vi "Scan Calculations.vi"(0 "counter cluster in":T6, 1 "control flags in":T5, 2 "N spot tracker in":T2, 3 "scan specification in":T7={"z resolution (pixels)"=1000, "iterations per pixel"=28, "iterations per z-scan (=zres*iterperpixel)"=50, "x resolution (pixels)"=100, "y resolution (pixels)"=80, "number of z-lines per volume"=30, "number of repetitions (volumes)"=5, "Pockels cell voltage (bits)"=-1, "Vx center (bits)"=0, "Vy center (bits)"=0, "Vx amplitude (bits)"=40, "Vy amplitude (bits)"=0, "lines to delay between scan start and output"=1, "LSB has acquire control"=FALSE}, 4 "tracking settings":T9, 5 "3-axis PV tracking state in":T3, 6 "x-y phase shift (*2^16/2*pi)":u16=16384, 7 "min photons for update":u32=200, 8 "Tracking State Initializer":T1, 11 "stim buffer counts":u16=20) -> (10 "end scan":bool, 12 "trigger out":bool, 13 "kalman to host":cluster{"Kalman State":T4, "Kalman Update":bool}, 14 "counter cluster out":T6, 15 "control flags out":T5, 16 "N spot tracker out":T2, 17 "scan specification out":T7, 18 "DAC voltages":T8 {"pockels" max=4095 step=1; "y" max=4095 step=1; "x" max=4095 step=1}, 19 "3-axis PV tracking state out":T3={"x state"={"pos estimate"=0.0, "v estimate"=0.0, "weighted position error sum"=0.0, "photon count"=0, "transmit tick count"=0, "axis number"=0, "px (levels^2)"=0.0, "pxv (levels^2/ticks)"=0.0, "pv (levels^2/ticks^2)"=0.0, "vel diff (levels^2/ticks^3)"=0.0, "gx"=0.0, "rtwiddle"=0.0, "photon count ch0"=0, "photon count ch1"=0, "Dx - for pos only k-f"=0.0}, "y state"={"pos estimate"=0.0, "v estimate"=0.0, "weighted position error sum"=0.0, "photon count"=0, "transmit tick count"=0, "axis number"=1, "px (levels^2)"=0.0, "pxv (levels^2/ticks)"=0.0, "pv (levels^2/ticks^2)"=0.0, "vel diff (levels^2/ticks^3)"=0.0, "gx"=0.0, "rtwiddle"=0.0, "photon count ch0"=0, "photon count ch1"=0, "Dx - for pos only k-f"=0.0}, "z state"={"pos estimate"=0.0, "v estimate"=0.0, "weighted position error sum"=0.0, "photon count"=0, "transmit tick count"=0, "axis number"=2, "px (levels^2)"=0.0, "pxv (levels^2/ticks)"=0.0, "pv (levels^2/ticks^2)"=0.0, "vel diff (levels^2/ticks^3)"=0.0, "gx"=0.0, "rtwiddle"=0.0, "photon count ch0"=0, "photon count ch1"=0, "Dx - for pos only k-f"=0.0}})   [LabVIEW 2010]
uses:
  FPGA tracking/polar tracking settings.ctl
  common_typedefs/DAC_voltage_tagResonantr.ctl
  scan_specification_tagResonant.ctl
  counter_cluster_tagResonant.ctl
  FPGA tracking/kalman 3-axis state.ctl
  FPGA tracking/integrating single axis kalman state.ctl
  FPGA tracking/control flags.ctl
  FPGA tracking/kalman N spot state.ctl
  FPGA tracking/tracking state initializer.ctl
panel:
  out "checked out state number":u16
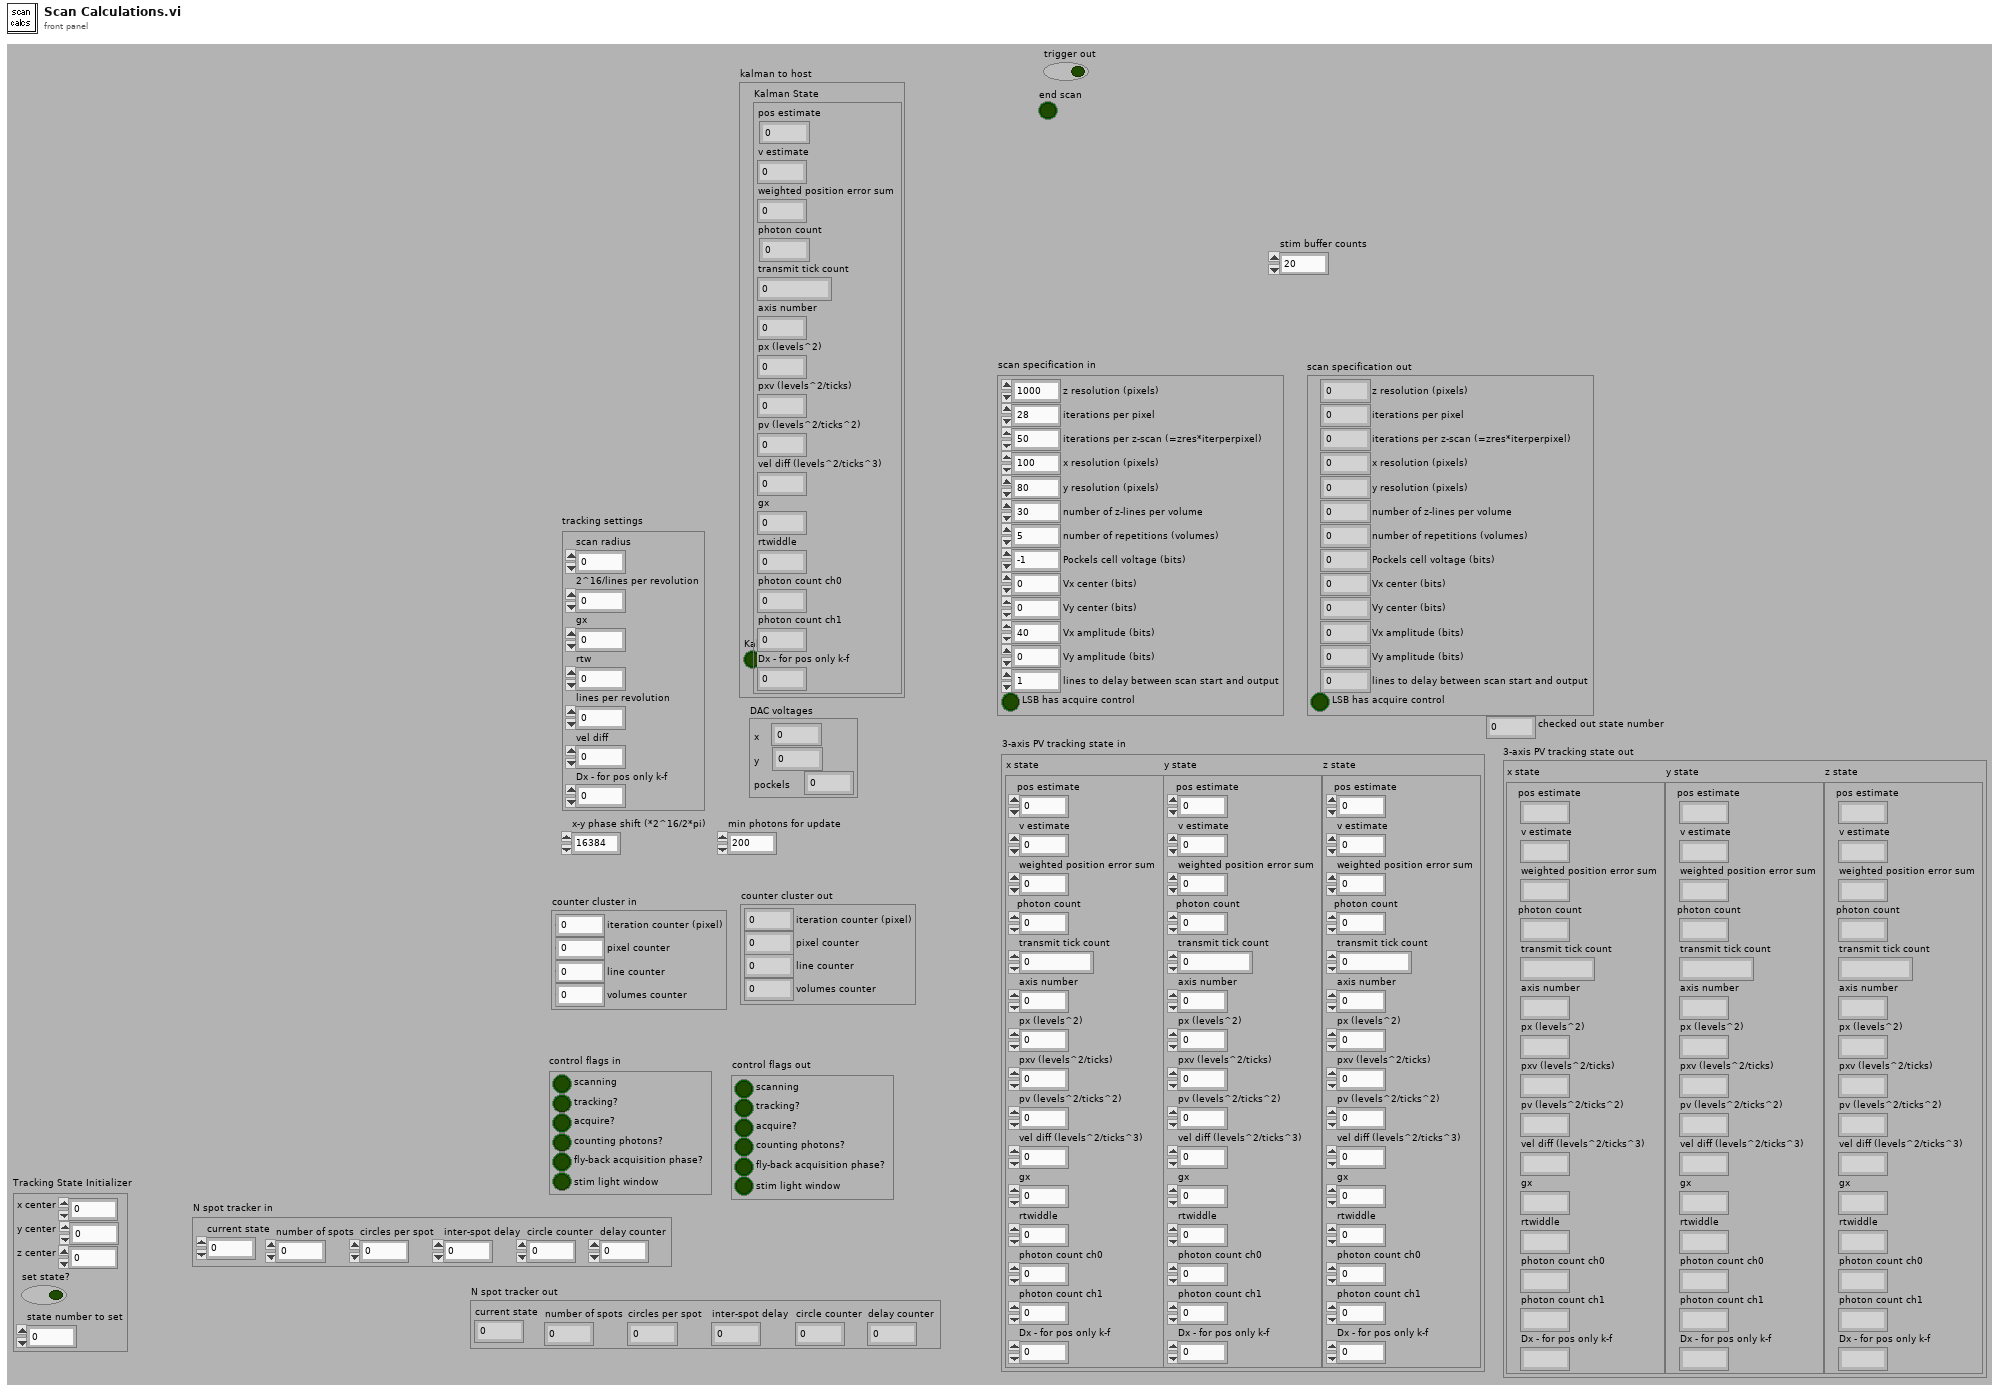
[diagram p1: front panel]
types:
  T1 = typedef "tracking state initializer.ctl" = cluster{"x center":i16, "y center":i16, "z center":i16, "set state?":bool, "state number to set":u16}
  T2 = typedef "kalman N spot state.ctl" = cluster{"current state":u8, "number of spots":u8, "circles per spot":u8, "inter-spot delay":u8, "circle counter":u8, "delay counter":u8}
  T3 = typedef "kalman 3-axis state.ctl" = cluster{"x state":T4, "y state":T4, "z state":T4}
  T4 = typedef "integrating single axis kalman state.ctl" = cluster{"pos estimate":fxp<+/-,32,16>, "v estimate":fxp<+/-,16,0>, "weighted position error sum":fxp<+/-,32,32>, "photon count":u32, "transmit tick count":u32, "axis number":u8, "px (levels^2)":fxp<+,32,19>, "pxv (levels^2/ticks)":fxp<+,32,2>, "pv (levels^2/ticks^2)":fxp<+,32,-14>, "vel diff (levels^2/ticks^3)":fxp<+,24,-22>, "gx":fxp<+,16,8>, "rtwiddle":fxp<+,16,26>, "photon count ch0":u32, "photon count ch1":u32, "Dx - for pos only k-f":fxp<+,32,19>}
  T5 = typedef "control flags.ctl" = cluster{"scanning":bool, "tracking?":bool, "acquire?":bool, "counting photons?":bool, "fly-back acquisition phase?":bool, "stim light window":bool}
  T6 = typedef "counter_cluster_tagResonant.ctl" = cluster{"iteration counter (pixel)":u16, "pixel counter":u16, "line counter":i16, "volumes counter":u16}
  T7 = typedef "scan_specification_tagResonant.ctl" = cluster{"z resolution (pixels)":u16, "iterations per pixel":u16, "iterations per z-scan (=zres*iterperpixel)":u16, "x resolution (pixels)":u16, "y resolution (pixels)":u16, "number of z-lines per volume":u16, "number of repetitions (volumes)":i32, "Pockels cell voltage (bits)":i16, "Vx center (bits)":i16, "Vy center (bits)":i16, "Vx amplitude (bits)":i16, "Vy amplitude (bits)":i16, "lines to delay between scan start and output":u16, "LSB has acquire control":bool}
  T8 = typedef "DAC_voltage_tagResonantr.ctl" = cluster{"x":i16, "y":i16, "pockels":i16}
  T9 = typedef "polar tracking settings.ctl" = cluster{"scan radius":u16, "2^16/lines per revolution":u16, "gx":fxp<+,16,8>, "rtw":fxp<+,16,26>, "lines per revolution":u8, "vel diff":fxp<+,24,-22>, "Dx - for pos only k-f":fxp<+,32,19>}
  T10 = cluster{"update x":bool, "update y":bool, "update z":bool}
  T11 = cluster{"counts per cycle":u16, "num triggers":u32, "fb end":u16, "fb start":u16, "ff start":u16, "ff end":u16}
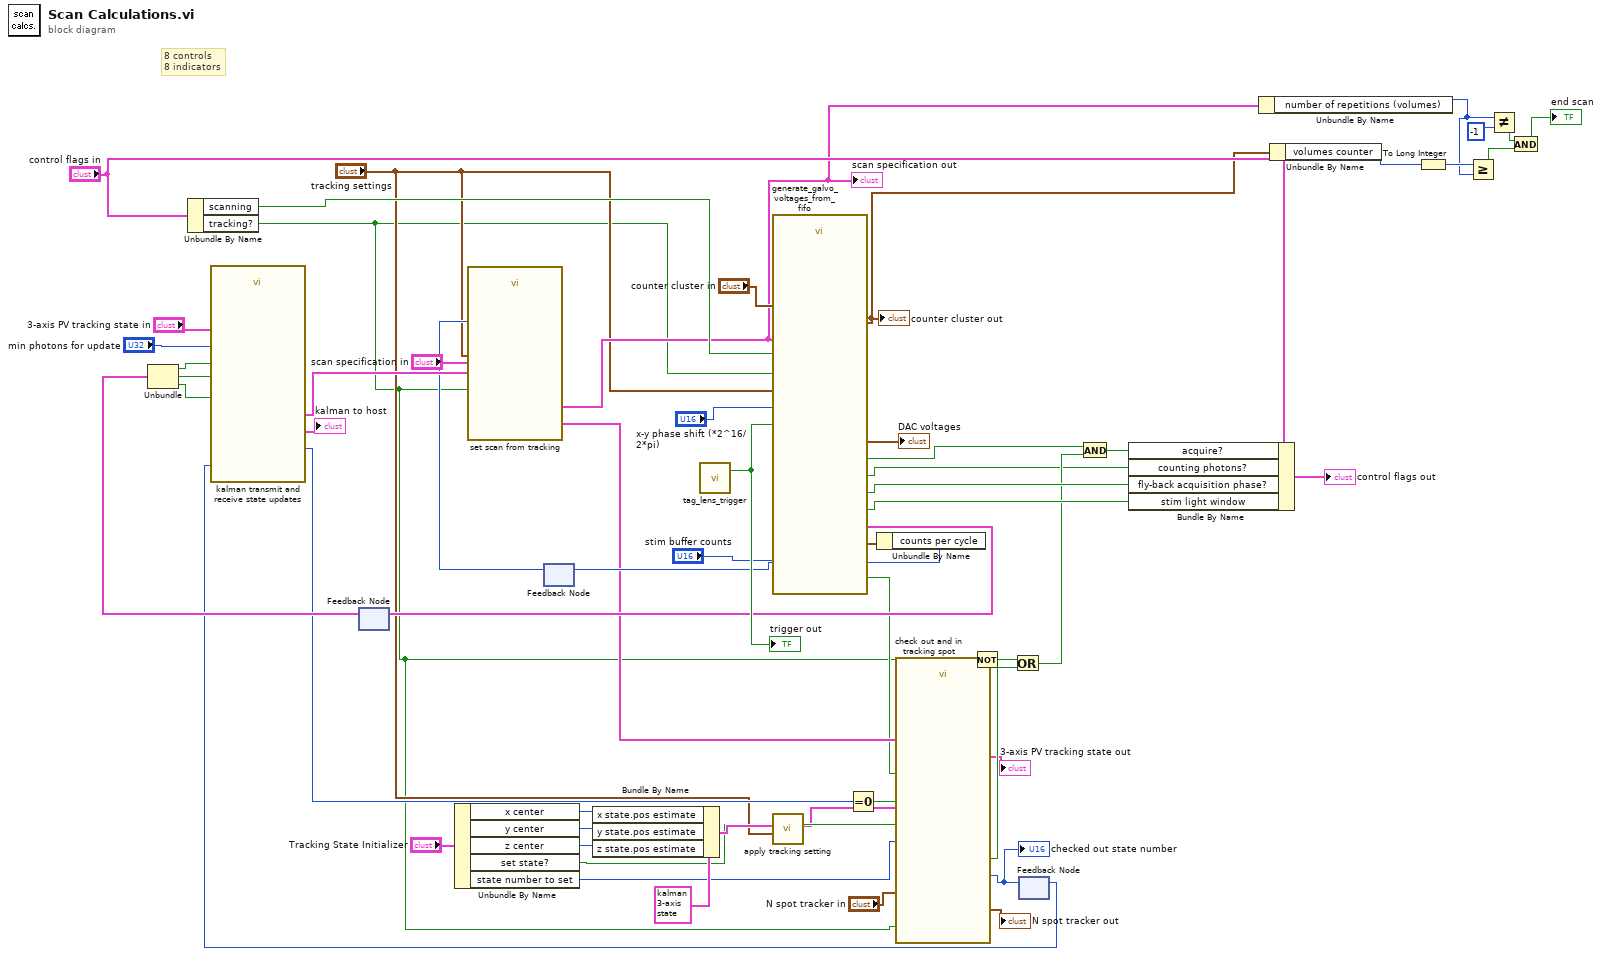
[diagram p0: block diagram]
diagram:
  # "8 controls\n8 indicators"
  n1 = Unbundle By Name("control flags in") -> ("scanning"=w39:bool, "tracking?"=w1:bool)
  n2 = feedback #1() -> (w46:T10)  [unwired: 1 in]
  n3 = Unbundle(w46) -> ("update x"=w50:bool, "update y"=w49:bool, "update z"=w48:bool)
  n4 = Unbundle By Name("Tracking State Initializer") -> ("x center"=w14:i16, "y center"=w13:i16, "z center"=w12:i16, "set state?"=w9:bool, "state number to set"=w8:u16)
  n5 = feedback #2() -> (w51:u16)  [unwired: 1 in]
  n6 = Bundle By Name(cluster=T3 {"x state"={"pos estimate"=0.0, "v estimate"=0.0, "weighted position error sum"=0.0, "photon count"=0, "transmit tick count"=0, "axis number"=0, "px (levels^2)"=0.0, "pxv (levels^2/ticks)"=0.0, "pv (levels^2/ticks^2)"=0.0, "vel diff (levels^2/ticks^3)"=0.0, "gx"=0.0, "rtwiddle"=0.0, "photon count ch0"=0, "photon count ch1"=0, "Dx - for pos only k-f"=0.0}, "y state"={"pos estimate"=0.0, "v estimate"=0.0, "weighted position error sum"=0.0, "photon count"=0, "transmit tick count"=0, "axis number"=1, "px (levels^2)"=0.0, "pxv (levels^2/ticks)"=0.0, "pv (levels^2/ticks^2)"=0.0, "vel diff (levels^2/ticks^3)"=0.0, "gx"=0.0, "rtwiddle"=0.0, "photon count ch0"=0, "photon count ch1"=0, "Dx - for pos only k-f"=0.0}, "z state"={"pos estimate"=0.0, "v estimate"=0.0, "weighted position error sum"=0.0, "photon count"=0, "transmit tick count"=0, "axis number"=2, "px (levels^2)"=0.0, "pxv (levels^2/ticks)"=0.0, "pv (levels^2/ticks^2)"=0.0, "vel diff (levels^2/ticks^3)"=0.0, "gx"=0.0, "rtwiddle"=0.0, "photon count ch0"=0, "photon count ch1"=0, "Dx - for pos only k-f"=0.0}} ("set state value"), "x state.pos estimate"=w14, "y state.pos estimate"=w13, "z state.pos estimate"=w12) -> (w11:T3)
  n7 = call "tag_lens_trigger.vi"() -> ("trigger out"=w55:bool)  [unwired: 2 in]
  "trigger out" <- w55
  n8 = call "apply tracking setting.vi"("tracking settings"="tracking settings", "tracking state in"=w11) -> ("tracking state out"=w7:T3)  [unwired: 9 in]
  n9 = Not(x=w1) -> (.not. x?=w20:bool)
  n10 = feedback #3() -> (w6:u8)  [unwired: 1 in]
  n11 = call "kalman transmit and receive state updates.vi"("current state"=w6, "min photons to update"="min photons for update", "update z"=w48, "update y"=w49, "update x"=w50, "3-axis PV tracking state"="3-axis PV tracking state in") -> ("num kalmans queued"=w25:u16, "3-axis PV tracking state out"=w58:T3, "kalman to host"=→"kalman to host":cluster{"Kalman State":T4, "Kalman Update":bool})  [unwired: 1 in, 2 out]
  n12 = call "set scan from tracking.vi"("tracking?"=w1, "counts per cycle"=w51, "tracking settings"="tracking settings", "tracking state in"=w58, "scan specification"="scan specification in") -> ("tracking state out"=w26:T3, "scan specification out"=w28:T7)  [unwired: 5 in]
  "scan specification out" <- w28
  n13 = call "generate_galvo_voltages_from_fifo.vi"("resonant trigger"=w55, "counter cluster in"="counter cluster in", "stim buffer counts"="stim buffer counts", "tracking settings"="tracking settings", "scan specification"=w28, "scanning"=w39, "tracking"=w1, "x-y phase shift (*2^16/2*pi)"="x-y phase shift (*2^16/2*pi)") -> ("stim light window"=w40:bool, "trigger diagnostics"=w53:T11, "update tracking?"=w47:T10, "counting photons?"=w2:bool, "DAC voltages"=→"DAC voltages":T8, "counter cluster out"=w29:T6, "new circle"=w23:bool, "fly-back acquisition phase?"=w41:bool, "acquire?"=w3:bool)  [unwired: 3 in]
  "counter cluster out" <- w29
  n14 = feedback-in #1(w47) -> ()
  n15 = Equal To 0?(x=w25) -> (x = 0?=w24:bool)
  n16 = Unbundle By Name(w53) -> ("counts per cycle"=w52:u16)
  n17 = feedback-in #2(w52) -> ()
  n18 = call "check out and in tracking spot.vi"("N spot tracker in"="N spot tracker in", "set state?"=w9, "tracking?"=w1, "tracking state in"=w26, "new circle"=w23, "permission to swap states"=w24, "set state value"=w7, "state number to set"=w8) -> ("N spot tracker out"=→"N spot tracker out":T2, "tracking state out"=→"3-axis PV tracking state out":T3, "checked out state number"=w5:u8, "use photons to track"=w22:bool)  [unwired: 4 in]
  "checked out state number" <- w5
  n19 = Or(x=w20, y=w22) -> (x .or. y?=w21:bool)
  n20 = feedback-in #3(w5) -> ()
  n21 = And(x=w3, y=w21) -> (x .and. y?=w4:bool)
  n22 = Bundle By Name(cluster="control flags in", "acquire?"=w4, "counting photons?"=w2, "fly-back acquisition phase?"=w41, "stim light window"=w40) -> (→"control flags out":T5)
  n23 = Unbundle By Name(w28) -> ("number of repetitions (volumes)"=w31:i32)
  n24 = Unbundle By Name(w29) -> ("volumes counter"=w33:u16)
  n25 = To Long Integer(number=w33) -> (32bit integer=w32:i32)
  n26 = Greater Or Equal?(x=w32, y=w31) -> (x >= y?=w35:bool)
  n27 = Not Equal?(x=w31, y=-1) -> (x != y?=w34:bool)
  n28 = And(x=w34, y=w35) -> (x .and. y?=→"end scan":bool)
